vi "DAQ Loop.vi"(8 "error in":errorcluster, 10 "Queues":T1, 11 "Notifiers":T2) -> (0 "error out":errorcluster)   [LabVIEW 2014, in "DAQ.lvlib"]
uses:
  DAQ.lvlib
  support/Message Queue/Message Queue.lvlib
  TypeDefs/DAQ data.ctl
  <vilib>/ErrorRing/Error Ring.xnode
  PLC/PLC.lvlib
  <vilib>/Utility/error.llb/Error Cluster From Error Code.vi
  Support/Global names.vi
  Support/Message Queue/Message Cluster.ctl
  Support/Notifiers/Notifiers.ctl
  Support/Notifiers/Notifiers.lvlib
  Support/Message Queue/All Message Queues.ctl
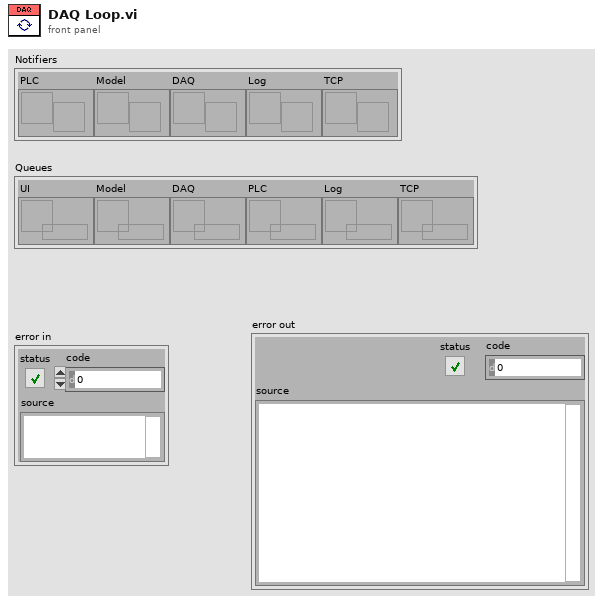
[diagram p1: front panel]
types:
  T1 = typedef "Message Queue.lvlib/All Message Queues.ctl" = cluster{"UI":refnum<queue>, "Model":refnum<queue>, "DAQ":refnum<queue>, "PLC":refnum<queue>, "Log":refnum<queue>, "TCP":refnum<queue>}
  T2 = typedef "Notifiers.lvlib/Notifiers.ctl" = cluster{"PLC":refnum<notifier>, "Model":refnum<notifier>, "DAQ":refnum<notifier>, "Log":refnum<notifier>, "TCP":refnum<notifier>}
  T3 = typedef "DAQ.lvlib/DAQ data.ctl" = cluster{"Power switch (DI)":cluster{"Channel":tag, "Data":bool}, "Dispose barrel (DI)":cluster{"Channel":tag, "Data":bool}, "Pump status (DO)":cluster{"Channel":tag, "Data":bool}, "Barrel position (AI)":cluster{"Channel":tag, "Data":dbl}}
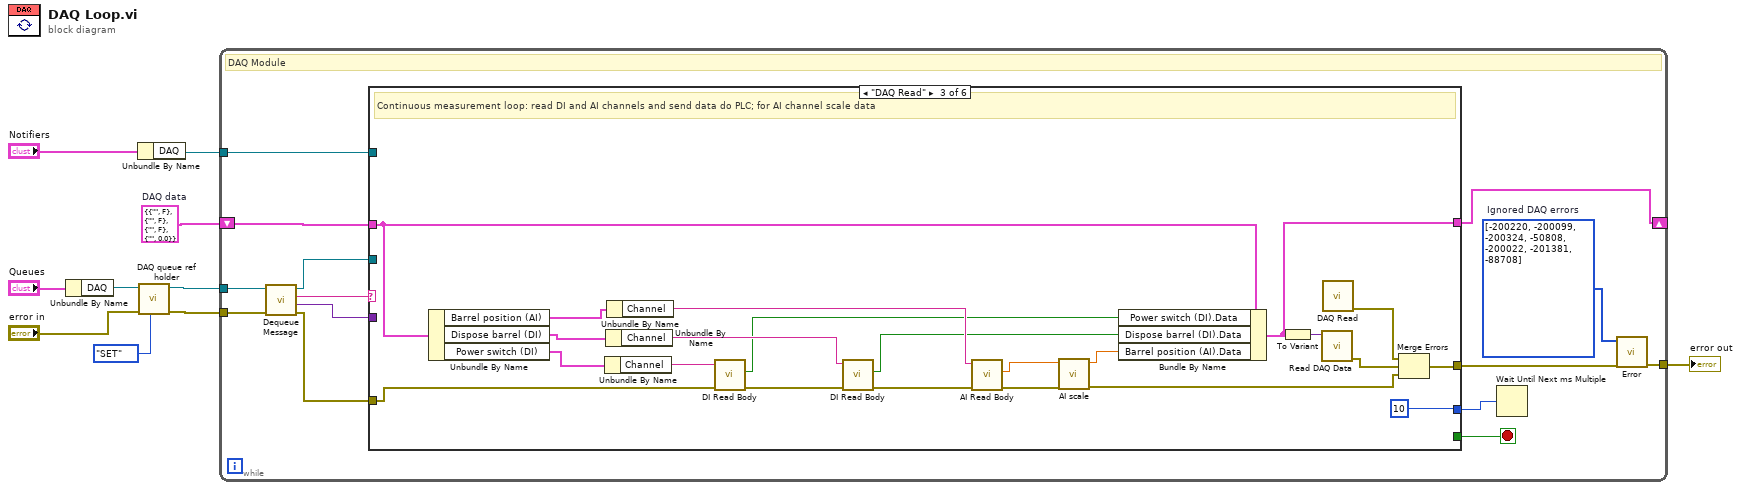
[diagram p0: block diagram]
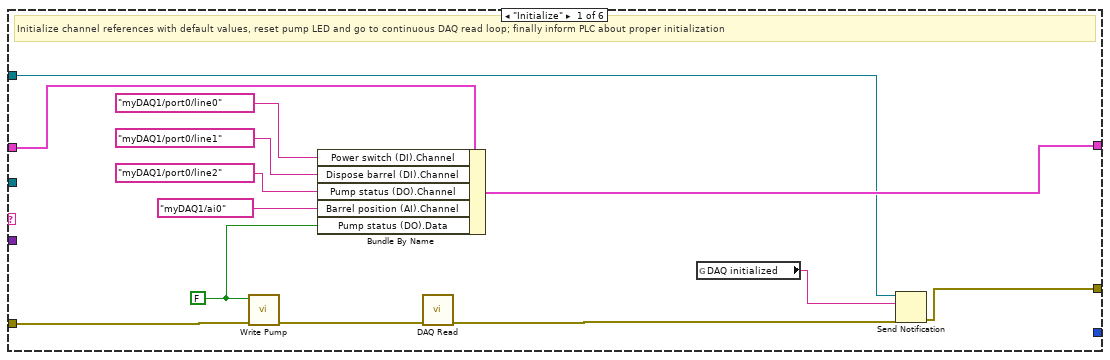
[diagram p2: hidden frame]
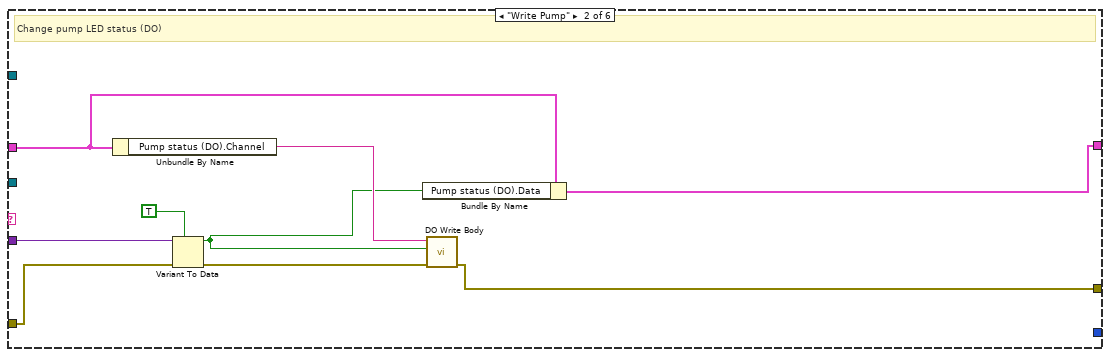
[diagram p3: hidden frame]
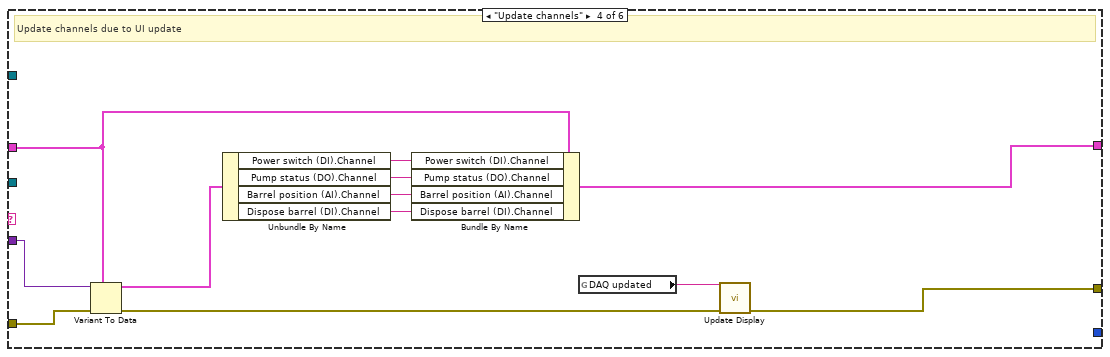
[diagram p4: hidden frame]
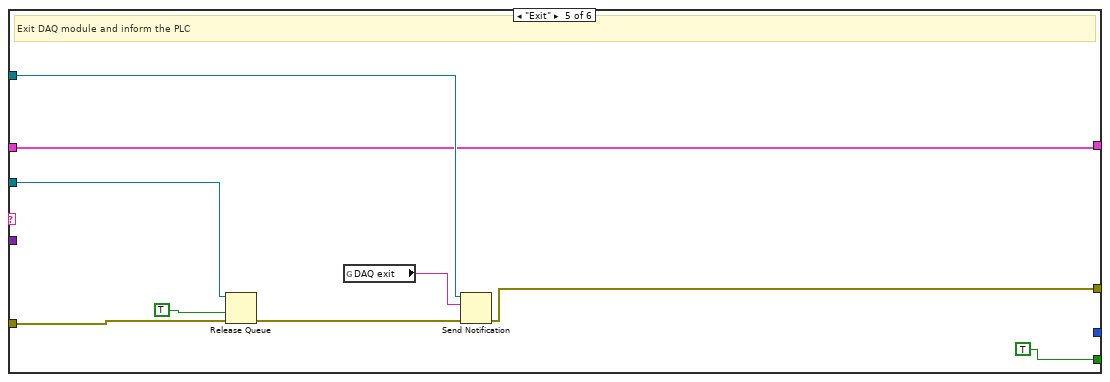
[diagram p5: hidden frame]
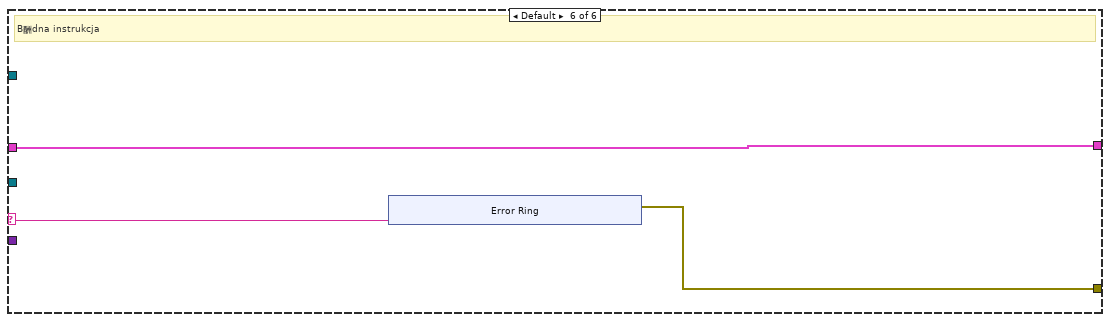
[diagram p6: hidden frame]
diagram:
  w10 = T3 {"Power switch (DI)"={"Channel"="", "Data"=FALSE}, "Dispose barrel (DI)"={"Channel"="", "Data"=FALSE}, "Pump status (DO)"={"Channel"="", "Data"=FALSE}, "Barrel position (AI)"={"Channel"="", "Data"=0.0}}  # DAQ data
  n1 = Unbundle By Name("Queues") -> ("DAQ"=w5:refnum<queue>)
  n2 = Unbundle By Name("Notifiers") -> ("DAQ"=w6:refnum<notifier>)
  n3 = call "DAQ queue ref holder.vi"("Action"=enum16{"GET", "SET"}."SET", "error in"="error in", "Message Queue In"=w5) -> ("error out"=w3:errorcluster, "Input Message Queue"=w4:refnum<queue>)  [unwired: 7 in]
  n4 = while {
    tunnel: w3 -> [w24]
    tunnel: w4 -> [w12]
    tunnel: w6 -> [w20]
    shift-right: [w19] -> _
    shift-left: w10 -> [w17]
    tunnel: [w15] -> w8
    stop <- w21 stop-if-true
    w11 = i32[] [-200220, -200099, -200324, -50808, -200022, -201381, -88708]  # Ignored DAQ errors
    # "DAQ Module"
    n5 = call "Dequeue Message.vi"("error in (no error)"=w24, "Message Queue"=w12) -> ("error out"=w23:errorcluster, "Message Data"=w22:variant, "Message"=w13:string, "dup Message Queue"=w14:refnum<queue>)  [unwired: 6 in]
    n6 = case shown="\"DAQ Read\"" w13 {
      selector: w13 -> [_ _ _ _ _ w91]
      tunnel: w23 -> [w30 w46 w55 w79 w83 _]
      tunnel: [w36 w38 w50 w71 w82 w90] -> w16
      tunnel: w22 -> [_ w45 _ w80 _ _]
      tunnel: [_ _ _ _ TRUE _] -> w21
      tunnel: w14 -> [_ _ _ _ w89 _]
      tunnel: w20 -> [w28 _ _ _ w88 _]
      tunnel: w17 -> [w35 w42 w65 w78 w84 w92]
      tunnel: [w34 w44 w59 w73 w84 w92] -> w19
      tunnel: [_ _ u32 10 ("millisecond multiple") _ _ _] -> w18
      frame "Initialize" {
        w27 = FALSE
        # "Initialize channel references with default values, reset pump LED and go to continuous DAQ read loop; finally inform PLC about proper initialization"
        n7 = call "Write Pump.vi"("error in"=w30, "Pump state"=w27) -> ("error out"=w29:errorcluster)  [unwired: 9 in]
        n8 = Bundle By Name(cluster=w35, "Power switch (DI).Channel"=tag "myDAQ1/port0/line0", "Dispose barrel (DI).Channel"=tag "myDAQ1/port0/line1" ("Power switch (DI).Channel"), "Pump status (DO).Channel"=tag "myDAQ1/port0/line2" ("Power switch (DI).Channel"), "Barrel position (AI).Channel"=tag "myDAQ1/ai0", "Pump status (DO).Data"=w27) -> (w34:T3)
        n9 = call "DAQ Read.vi"("error in"=w29) -> ("error out"=w26:errorcluster)  [unwired: 10 in]
        n10 = global read "Global names.vi" "DAQ initialized"() -> (w25:string)
        n11 = Send Notification(notification=w25, notifier=w28, error in (no error)=w26) -> (error out=w36:errorcluster)  [unwired: 1 out]
      }
      frame "Write Pump" {
        # "Change pump LED status (DO)"
        n12 = Unbundle By Name(w42) -> ("Pump status (DO).Channel"=w43:tag)
        n13 = Variant To Data(error in=w46, type=TRUE, Variant=w45) -> (data=w40:bool, error out=w39:errorcluster)
        n14 = Bundle By Name(cluster=w42, "Pump status (DO).Data"=w40) -> (w44:T3)
        n15 = call "DO Write Body.vi"("error in"=w39, "data"=w40, "Channel"=w43) -> ("error out"=w38:errorcluster)  [unwired: 6 in]
      }
      frame "DAQ Read" {
        # "Continuous measurement loop: read DI and AI channels and send data do PLC; for AI channel scale data"
        n16 = Unbundle By Name(w65) -> ("Barrel position (AI)"=w52:cluster{"Channel":tag, "Data":dbl}, "Dispose barrel (DI)"=w53:cluster{"Channel":tag, "Data":bool}, "Power switch (DI)"=w54:cluster{"Channel":tag, "Data":bool})
        n17 = Unbundle By Name(w54) -> ("Channel"=w64:tag)
        n18 = Unbundle By Name(w53) -> ("Channel"=w63:tag)
        n19 = Unbundle By Name(w52) -> ("Channel"=w62:tag)
        n20 = call "DI Read Body.vi"("error in"=w55, "Channel"=w64) -> ("error out"=w68:errorcluster, "data"=w57:bool)  [unwired: 6 in]
        n21 = call "DI Read Body.vi"("error in"=w68, "Channel"=w63) -> ("error out"=w67:errorcluster, "data"=w58:bool)  [unwired: 6 in]
        n22 = call "AI Read Body.vi"("error in"=w67, "Channel"=w62) -> ("error out"=w51:errorcluster, "data"=w66:dbl)  [unwired: 6 in]
        n23 = call "AI scale.vi"("error in"=w51, "Data in"=w66) -> ("error out"=w47:errorcluster, "Data out"=w61:dbl)  [unwired: 8 in]
        n24 = Bundle By Name(cluster=w65, "Power switch (DI).Data"=w57, "Dispose barrel (DI).Data"=w58, "Barrel position (AI).Data"=w61) -> (w59:T3)
        n25 = To Variant(anything=w59) -> (Variant=w56:variant)
        n26 = call "Read DAQ Data.vi"("Message Data"=w56) -> ("error out"=w48:errorcluster)  [unwired: 10 in]
        n27 = call "DAQ Read.vi"() -> ("error out"=w49:errorcluster)  [unwired: 11 in]
        n28 = Merge Errors(w49, w48, w47) -> (w50:errorcluster)
      }
      frame "Update channels" {
        # "Update channels due to UI update"
        n29 = Variant To Data(error in=w79, type=w78, Variant=w80) -> (data=w70:T3, error out=w72:errorcluster)
        n30 = Unbundle By Name(w70) -> ("Power switch (DI).Channel"=w77:tag, "Pump status (DO).Channel"=w76:tag, "Barrel position (AI).Channel"=w75:tag, "Dispose barrel (DI).Channel"=w74:tag)
        n31 = Bundle By Name(cluster=w78, "Power switch (DI).Channel"=w77, "Pump status (DO).Channel"=w76, "Barrel position (AI).Channel"=w75, "Dispose barrel (DI).Channel"=w74) -> (w73:T3)
        n32 = global read "Global names.vi" "DAQ updated"() -> (w69:string)
        n33 = call "Update Display.vi"("error in"=w72, "Message string"=w69) -> ("error out"=w71:errorcluster)  [unwired: 9 in]
      }
      frame "Exit" {
        # "Exit DAQ module and inform the PLC"
        n34 = Release Queue(queue=w89, force destroy? (F)=TRUE, error in (no error)=w83) -> (error out=w87:errorcluster)  [unwired: 2 out]
        n35 = global read "Global names.vi" "DAQ exit"() -> (w81:string)
        n36 = Send Notification(notification=w81, notifier=w88, error in (no error)=w87) -> (error out=w82:errorcluster)  [unwired: 1 out]
      }
      frame Default {
        # "B酬dna instrukcja"
        n37 = xnode "Error Ring"("parameter 0"=w91) -> ("error out"=w90:errorcluster)
      }
    }
    n38 = Wait Until Next ms Multiple(millisecond multiple=w18) -> ()  [unwired: 1 out]
    n39 = call "Error.vi"("error in"=w16, "Ignore Errors (Runtime)"=w11) -> ("error out"=w15:errorcluster)  [unwired: 9 in]
  }
  "error out" <- w8
